vi "Mpemba1_QPDcali.vi"() -> ()   [LabVIEW 2019]
uses:
  <vilib>/rvi/Emulation/niFpgaGetClockAttributes.vi
  <vilib>/rvi/Emulation/niFpgaSctlEmulationGetInTimedLoop.vi
  <vilib>/rvi/Emulation/niFpgaEmulationReportErrorSimple.vi
  <vilib>/rvi/eio/common/nirviEmuTemplateMethod_errors.vi
  <vilib>/rvi/Emulation/niFpgaCriticalErrorInLSC.vi
  <vilib>/rvi/eio/common/nirviEmuTemplatePropertySet_noerrors.vi
  <vilib>/rvi/Emulation/niFpgaProcessEmulError.vi
  <vilib>/rvi/occurrence/nirviWaitOnOccurrenceBase.vi
  <vilib>/rvi/Emulation/niFpgaEmulationIsFPGAContextNoSignature.vi
  <vilib>/rvi/errors/niFpgaSetErrorForExecOnDevCompSimple.vi
  <vilib>/rvi/eio/common/nirviEmuReportErrorAndStop.vi
  <vilib>/rvi/DataTransferAndStorage/Container/Common/niFpgaContainerGetUniqueNameForEmu.vi
  <vilib>/rvi/FIFO/Fifo_Resource/nirvififoEmulationSetSize.vi
  <vilib>/rvi/FIFO/Fifo_Resource/nirviFifoEmulationQueueMgr.vi
  <instcachedir>/0/nirviFifoEmulationQueueMgr_E5CAEC123FF24DC58D834DCA3CDAA9B5.lvgen/nirviFifoEmulationQueueMgr_E5CAEC123FF24DC58D834DCA3CDAA9B5_001.vi
  <vilib>/Utility/error.llb/Clear Errors.vi
  <vilib>/rvi/FIFO/Fifo_Resource/nirvififoEmulationCreateLock.vi
  <vilib>/rvi/FIFO/Fifo_Resource/nirvififoEmulationObtainLock.vi
  <vilib>/rvi/FIFO/Fifo_Resource/nirvififoEmulationReleaseLock.vi
  <vilib>/rvi/errors/nirviReportUnexpectedCaseInternalError.vi
  <vilib>/rvi/errors/nirviReportUnexpectedCaseInternalError (U32).vi
  <vilib>/rvi/interface/RandomDataEmulation/niFpgaRandomDataHandleErrors.vi
  <vilib>/rvi/FIFO/Fifo_Resource/nirvififoEmulationDetermineInputValidOut.vi
  <vilib>/eio/EIONode/EIONode.xnode
  <vilib>/eio/EIOPropertyNode/EIOPropertyNode.xnode
  <vilib>/rvi/DataTransferAndStorage/Container/XNode/niFpgaContainer.xnode
  <vilib>/rvi/FIFO/Fifo_Resource/nirvififoEmulationRead.vi
  <vilib>/rvi/interface/RandomDataEmulation/nirviRandomDataFpgaReadWriteTemplate.vi
  <vilib>/rvi/FIFO/Fifo_Resource/nirvififoEmulationWrite.vi
  <vilib>/rvi/eio/common/nirviEmuTemplatePropertyGet_errors.vi
  <vilib>/rvi/eio/common/nirviEmuTemplatePropertyGet_noerrors.vi
  <vilib>/rvi/eio/common/nirviEmuTemplatePropertySet_errors.vi
panel:
  in  "Flat potential\nboundary":sgl=2.0 format="%#_13g"
  out "Protocol\nnumber":u32
  out "Protocol \nloops":i16
  out "Trigger":bool
  in  "hw cal\ntime":sgl=50.0
  in  "AOD_AO4 2":sgl
  in  "AOD_AO0 2":sgl
  in  "V_offset":sgl
  in  "Calibration":T1
  in  "Bias":sgl
  out "Time":i32
  in  "Fmax":sgl
  out "Fx out/Xcorr":sgl
  out "Xpot":sgl format="%.2f"
  in  "Temp":i8(ring) items=["Cold", "Warm", "Hot"]
  in  "cdfnorm":sgl
  out "Saveloop":u32
  in  "Enum":T2(ring)
  in  "MobX(px/V)":sgl
  in  "1/Xcali":sgl
  in  "Feedback parameters":T3
  in  "DX":sgl
  in  "DW":cluster{"xm":sgl, "Eb":sgl, "Tau":sgl, "dE":sgl}={"xm"=0.0, "Eb"=0.0, "Tau"=50.0, "dE"=0.0}
  in  "Xmean":sgl
  in  "Calibration ON/OFF":bool
  in  "Frequency":u32=100000
  in  "wait time":sgl=35.0
  in  "Triangle wave":T4={"signal offset_X"=5.0, "Scale X"=0.0, "signal offset_Y"=5.0, "Scale Y"=0.0, "Phase Shift"=30}
  in  "Xoffset":sgl
  in  "Yoffset":sgl
  in  "sum_offset":sgl
  in  "Normalize signal":bool=TRUE
  in  "FB Time":u8=5 caption="Feedback loop time"
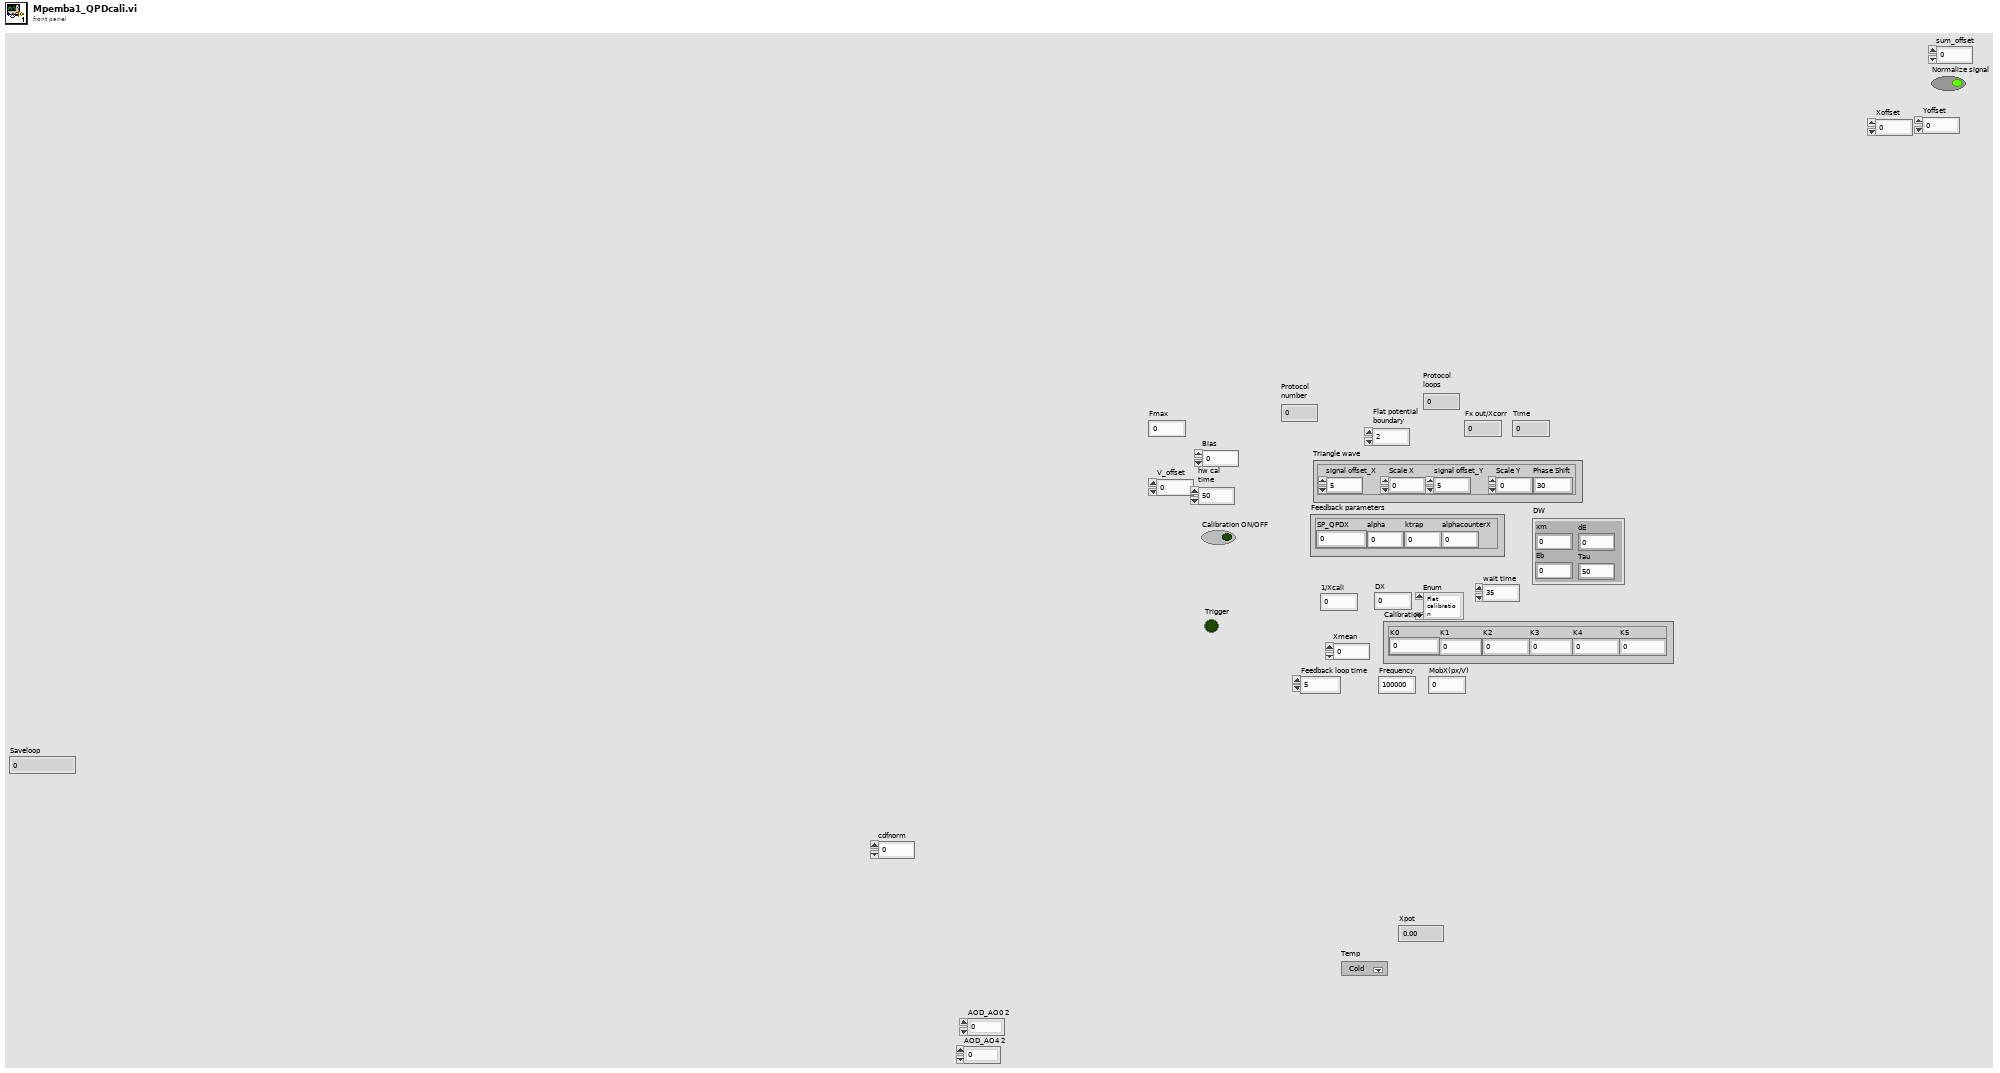
[diagram p1: front panel]
types:
  T1 = cluster{"K0":sgl, "K1":sgl, "K2":sgl, "K3":sgl, "K4":sgl, "K5":sgl}
  T2 = enum8{"Flat calibration", "Flat cal w drift corr", "No FB", "FB"}
  T3 = cluster{"SP_QPDX":sgl, "alpha":sgl, "ktrap":sgl, "alphacounterX":sgl}
  T4 = cluster{"signal offset_X":sgl, "Scale X":sgl, "signal offset_Y":sgl, "Scale Y":sgl, "Phase Shift":u32}
  T5 = enum8{"+/- 10 V", "+/- 5 V", "+/- 2 V", "+/- 1 V"}
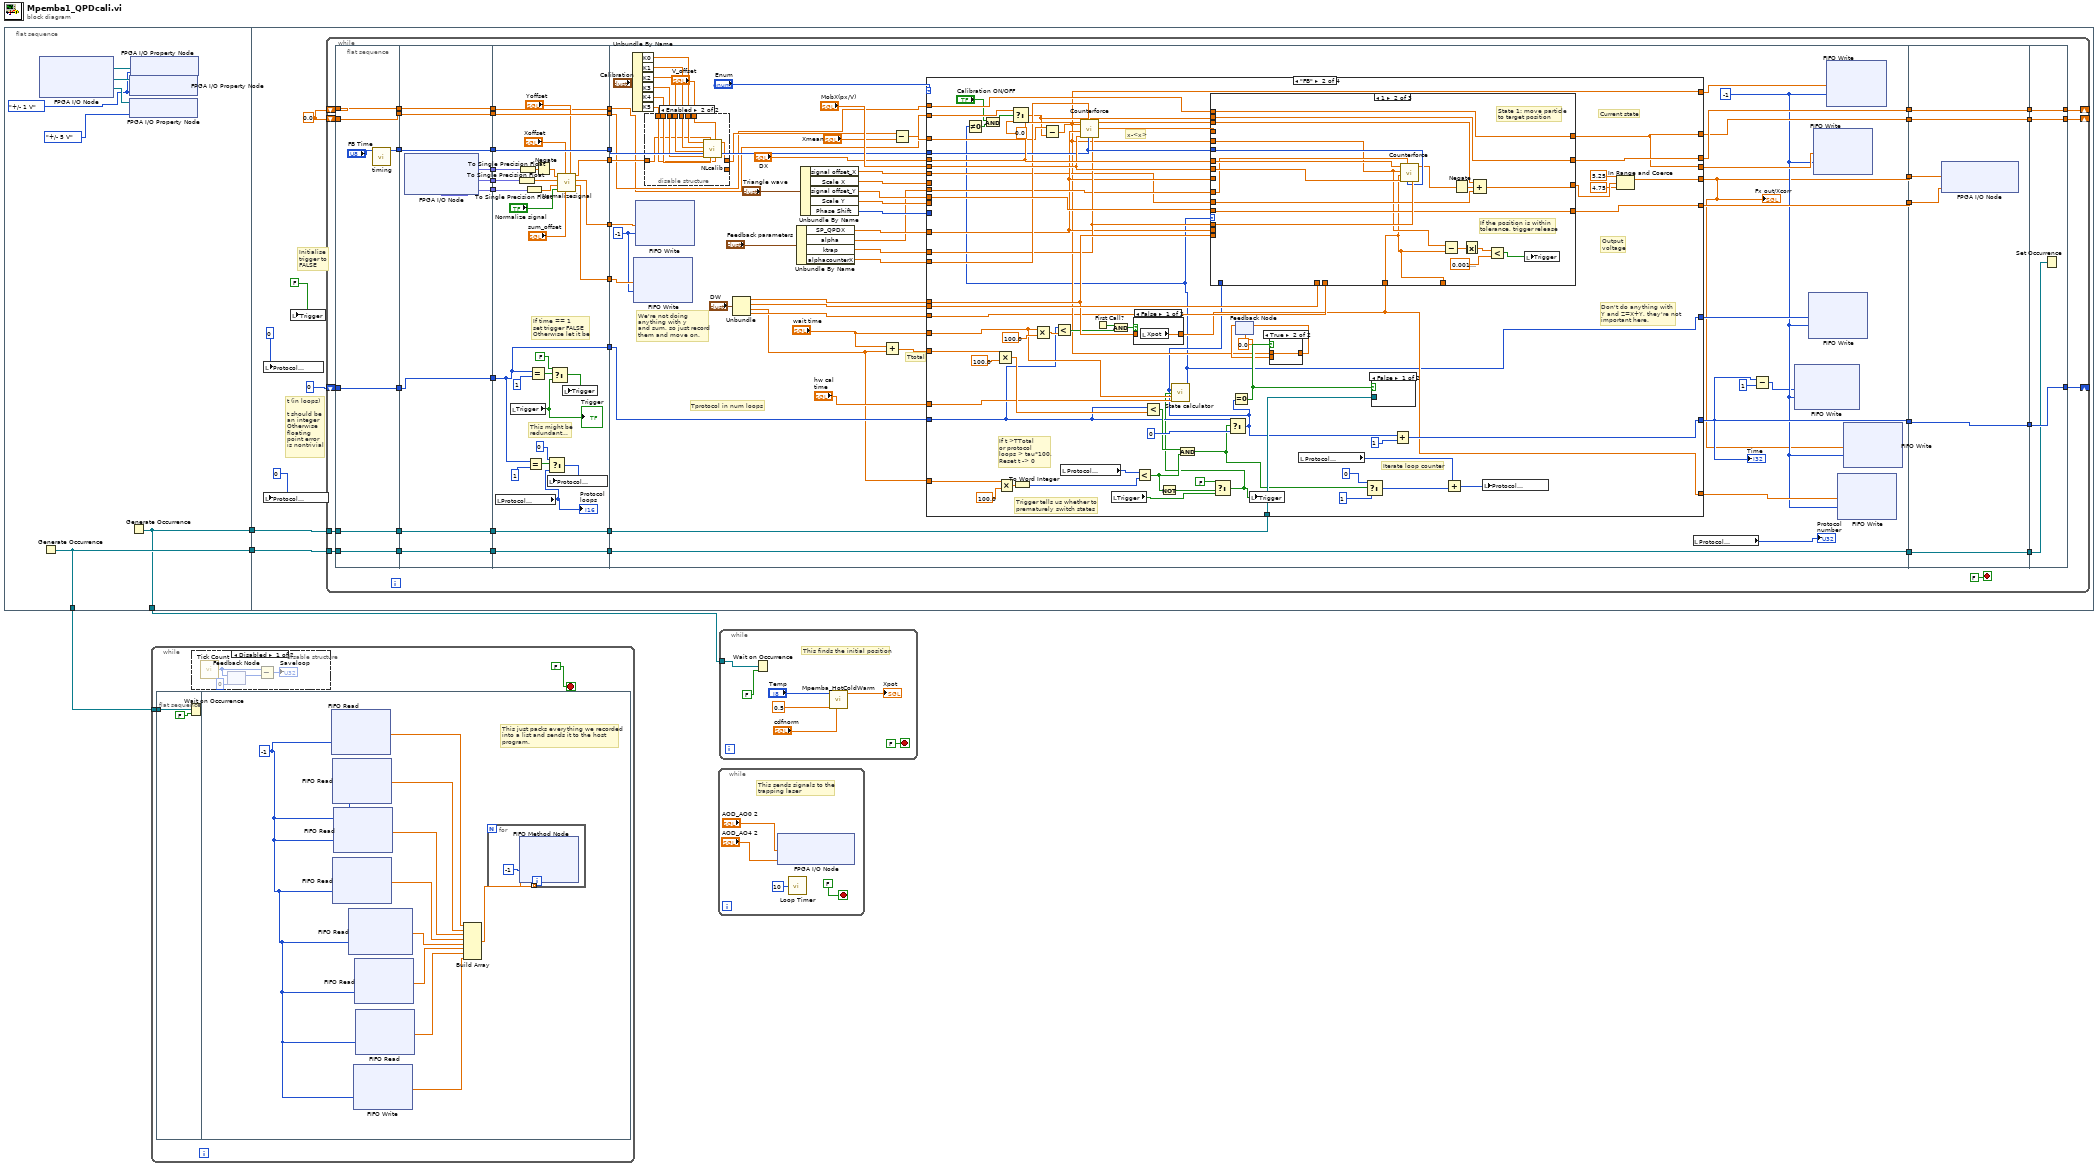
[diagram p0: block diagram]
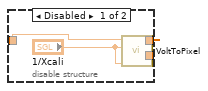
[diagram p2: hidden frame]
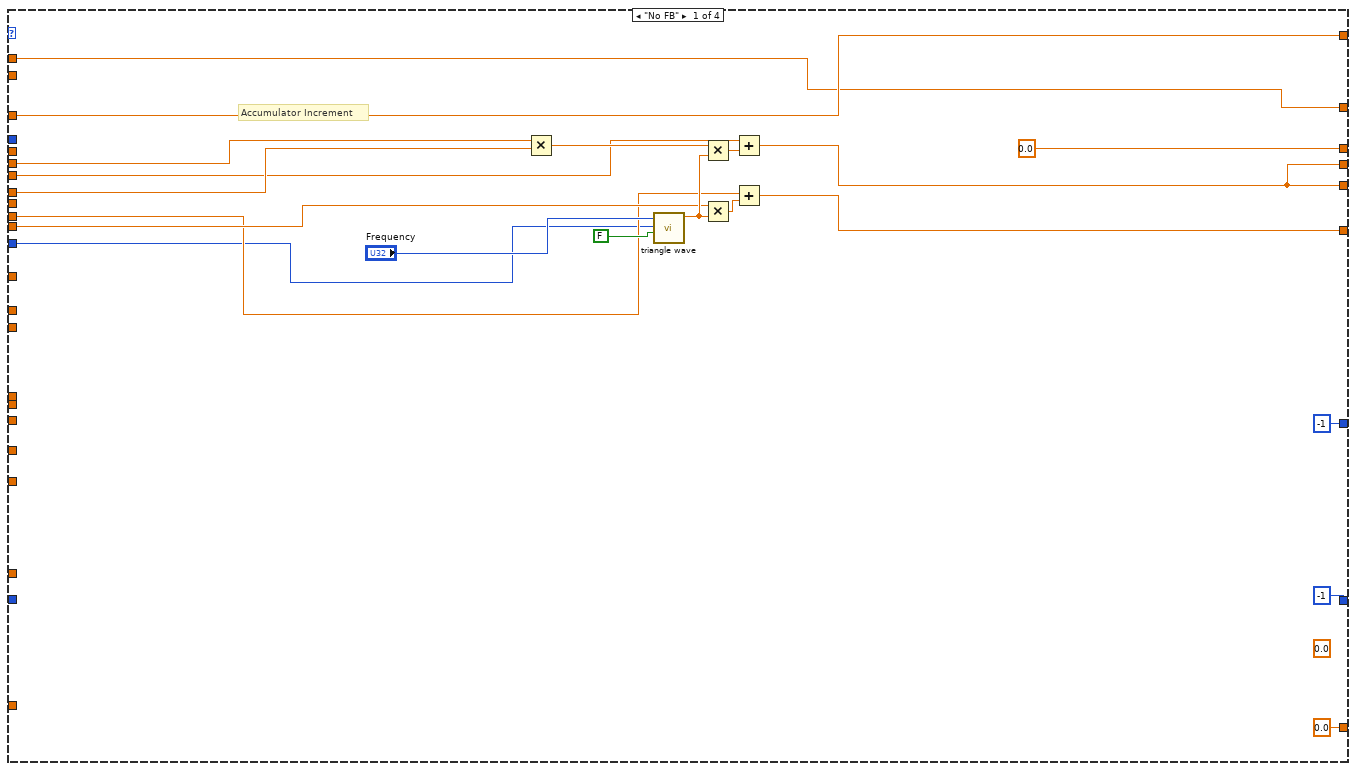
[diagram p3: hidden frame]
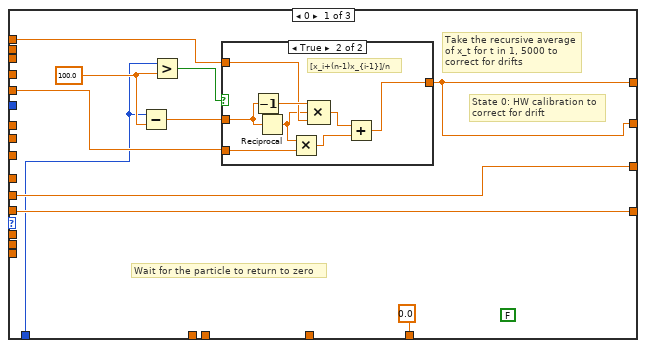
[diagram p4: hidden frame]
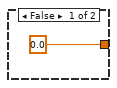
[diagram p5: hidden frame]
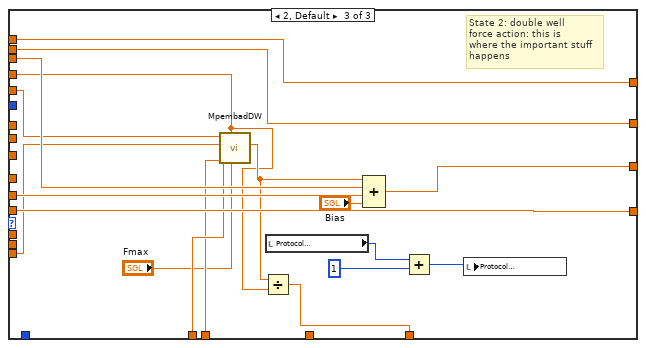
[diagram p6: hidden frame]
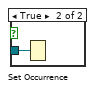
[diagram p7: hidden frame]
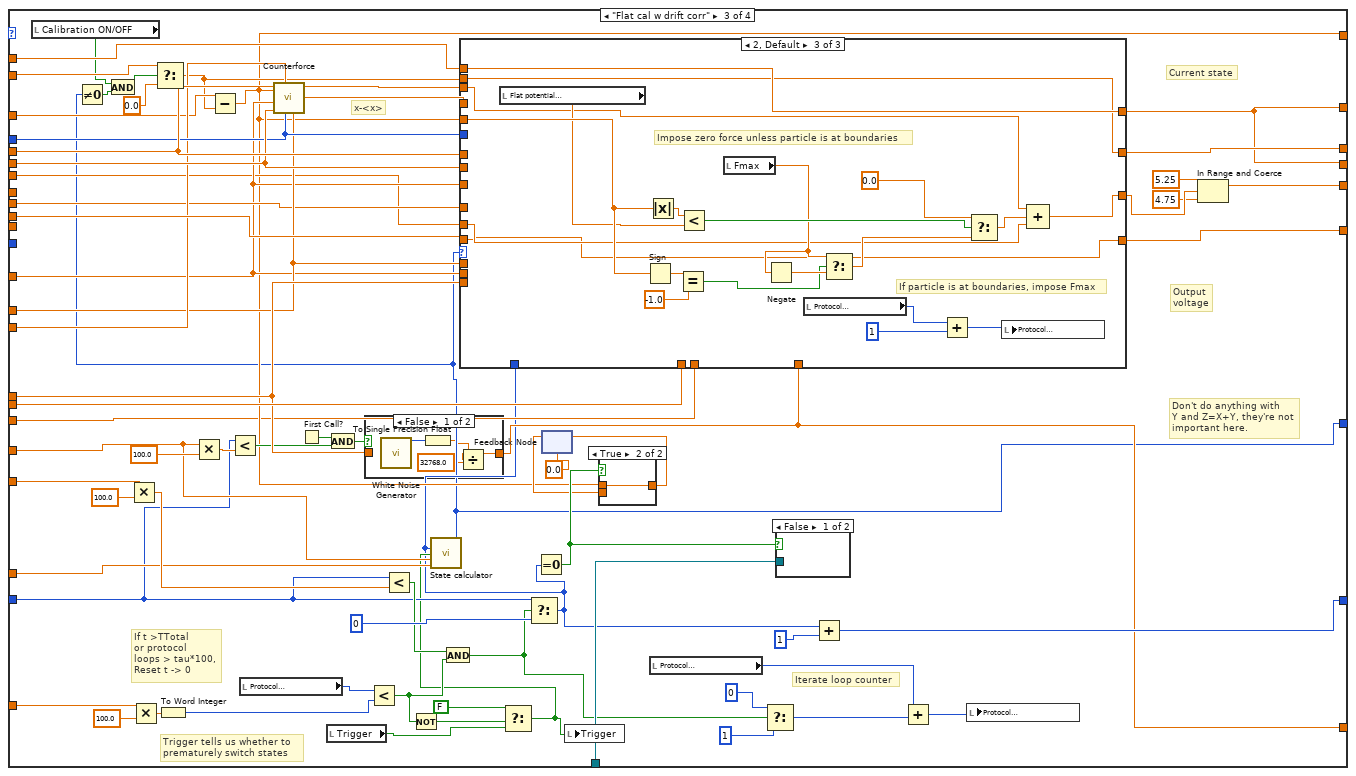
[diagram p10: hidden frame]
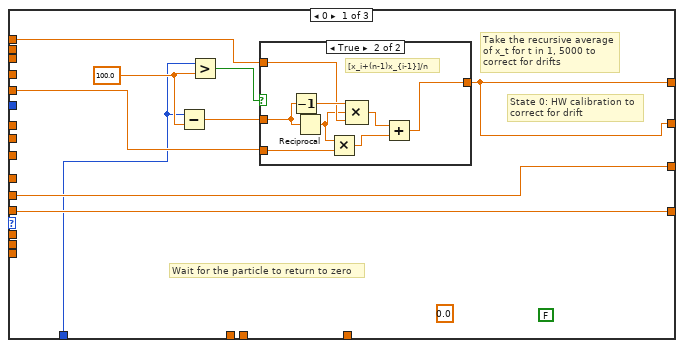
[diagram p11: hidden frame]
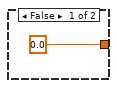
[diagram p12: hidden frame]
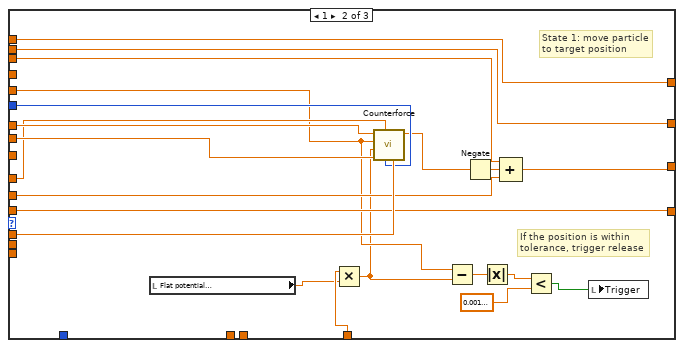
[diagram p13: hidden frame]
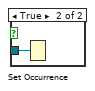
[diagram p14: hidden frame]
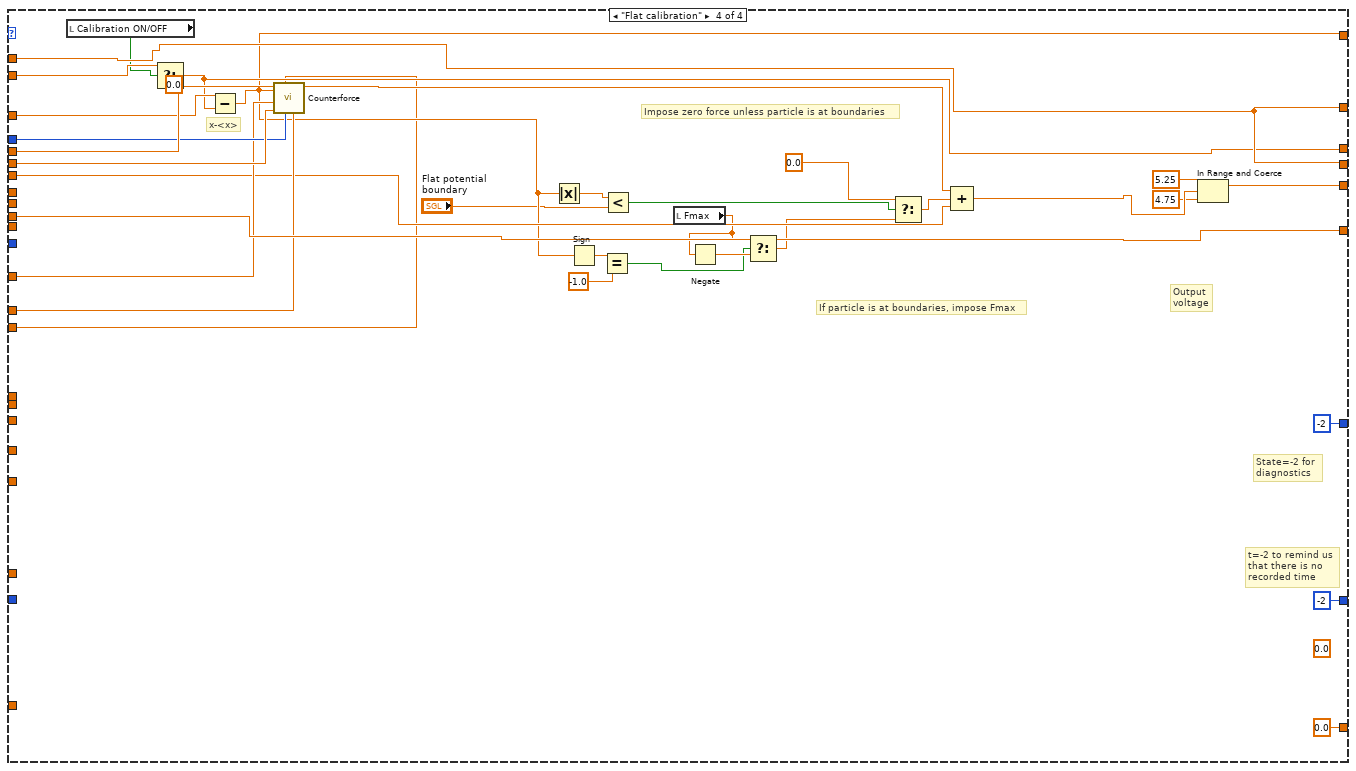
[diagram p17: hidden frame]
diagram:
  n1 = flat-sequence {
    tunnel: [w8] -> w2
    tunnel: [w7] -> w1
    tunnel: [w8] -> w4
    tunnel: [w7] -> w3
    tunnel: w2 -> [w18]
    tunnel: w1 -> [w17]
    frame #0 {
      w6 = T5."+/- 1 V" ("Voltage Range")
      n2 = xnode "FPGA I/O Node"() -> ("FPGA I/O Out"=w11:refnum<k21>, "FPGA I/O Out"=w9:refnum<k21>, "FPGA I/O Out"=w10:refnum<k21>)  [unwired: 3 in, 3 out]
      n3 = Generate Occurrence() -> (w8:refnum<k4>)
      n4 = xnode "FPGA I/O Property Node"("FPGA I/O In"=w9, "Voltage Range"=w6) -> ()  [unwired: 1 out]
      n5 = xnode "FPGA I/O Property Node"("FPGA I/O In"=w10, "Voltage Range"=T5."+/- 5 V") -> ()  [unwired: 1 out]
      n6 = Generate Occurrence() -> (w7:refnum<k4>)
      n7 = xnode "FPGA I/O Property Node"("FPGA I/O In"=w11, "Voltage Range"=w6) -> ()  [unwired: 1 out]
    }
    frame #1 {
      w16 = sgl 0.0
      # "t (in loops)\n\nt should be \nan integer\nOtherwise\nfloating\npoint error\nis nontrivial"
      # "Initialise\ntrigger to\nFALSE"
      n8 = local write "Protocol\nnumber"(u32 0 ("Protocol\nnumber")) -> ()
      n9 = local write "Protocol \nloops"(i16 0 ("Protocol loops")) -> ()
      n10 = local write "Trigger"(FALSE ("Trigger")) -> ()
      n11 = while {
        tunnel: w18 -> [w47]
        tunnel: w17 -> [w38]
        shift-right: [w35] -> _
        shift-left: w16 -> [w33]
        shift-right: [w28] -> _
        shift-left: w16 -> [w27]
        shift-right: [w19] -> _
        shift-left: i16 0 ("State") -> [w22]
        stop <- FALSE ("stop") stop-if-true
        n12 = flat-sequence {
          tunnel: [w67] -> w50
          tunnel: w47 -> [w66]
          tunnel: [w66] -> w46
          tunnel: [w65] -> w39
          tunnel: w38 -> [w65]
          tunnel: [w64] -> w34
          tunnel: w33 -> [w64]
          tunnel: w27 -> [w63]
          tunnel: [w63] -> w26
          tunnel: [w62] -> w23
          tunnel: w22 -> [w62]
          tunnel: [w77] -> w60
          tunnel: [w76] -> w58
          tunnel: [w75] -> w56
          tunnel: [w74] -> w51
          tunnel: w50 -> [w74]
          tunnel: w46 -> [w73]
          tunnel: [w73] -> w45
          tunnel: [w72] -> w40
          tunnel: w39 -> [w72]
          tunnel: w34 -> [w71]
          tunnel: [w71] -> w31
          tunnel: w26 -> [w70]
          tunnel: [w70] -> w25
          tunnel: w23 -> [w69]
          tunnel: [w69] -> w21
          tunnel: w60 -> [w91]
          tunnel: [w106] -> w59
          tunnel: w58 -> [w90]
          tunnel: [w105] -> w57
          tunnel: w56 -> [w89]
          tunnel: [w104] -> w55
          tunnel: [w107] -> w52
          tunnel: w51 -> [w107]
          tunnel: w45 -> [w103]
          tunnel: [w103] -> w44
          tunnel: [w102] -> w41
          tunnel: w40 -> [w102]
          tunnel: [w100] -> w32
          tunnel: w31 -> [w100]
          tunnel: w25 -> [w94]
          tunnel: [w94] -> w24
          tunnel: w21 -> [w78]
          tunnel: [w78] -> w20
          tunnel: w59 -> [w159]
          tunnel: w57 -> [w111]
          tunnel: w55 -> [w110]
          tunnel: [w112] -> w54
          tunnel: [w163] -> w53
          tunnel: w52 -> [w160]
          tunnel: [w119] -> w49
          tunnel: w44 -> [w152]
          tunnel: [w152] -> w42
          tunnel: w41 -> [w147]
          tunnel: [w115] -> w37
          tunnel: w32 -> [w145]
          tunnel: [w116] -> w30
          tunnel: w24 -> [w133]
          tunnel: w20 -> [w122]
          tunnel: w53 -> [w499]
          tunnel: w54 -> [w500]
          tunnel: w49 -> [w504]
          tunnel: [w504] -> w48
          tunnel: [w503] -> w43
          tunnel: w42 -> [w503]
          tunnel: w37 -> [w502]
          tunnel: [w502] -> w36
          tunnel: w30 -> [w501]
          tunnel: [w501] -> w29
          tunnel: w48 -> [w508]
          tunnel: [w508] -> w19
          tunnel: w43 -> [w507]
          tunnel: [w506] -> w35
          tunnel: w36 -> [w506]
          tunnel: w29 -> [w505]
          tunnel: [w505] -> w28
          frame #0 {
            n13 = call "timing.vi"("Feedback loop time"="FB Time") -> ("Feedback Loop time"=w67:u32)  [unwired: 10 in]
          }
          frame #1 {
            n14 = xnode "FPGA I/O Node"() -> ("Connector0/AI2"=w77:fxp<+/-,27,5>, "Connector0/AI4"=w76:fxp<+/-,27,5>, "Connector0/AI5"=w75:fxp<+/-,27,5>)  [unwired: 3 in, 3 out]
          }
          frame #2 {
            # "This might be\nredundant..."
            # "If time == 1\nset trigger FALSE\nOtherwise let it be"
            n15 = local read "Protocol \nloops"() -> (w80:i16)
            "Protocol \nloops" <- w80
            n16 = local read "Trigger"() -> (w84:bool)
            "Trigger" <- w84
            n17 = To Single Precision Float(number=w90) -> (single precision float=w96:sgl)
            n18 = To Single Precision Float(number=w91) -> (single precision float=w93:sgl)
            n19 = To Single Precision Float(number=w89) -> (single precision float=w95:sgl)
            n20 = Equal?(x=w78, y=i16 1) -> (x = y?=w82:bool)
            n21 = Equal?(x=w78, y=i16 1) -> (x = y?=w87:bool)
            n22 = Negate(x=w93) -> (-x=w92:sgl)
            n23 = Select(t=i16 0, s=w82, f=w80) -> (s? t:f=w81:i16)
            n24 = local write "Protocol \nloops"(w81) -> ()
            n25 = Select(t=FALSE, s=w87, f=w84) -> (s? t:f=w86:bool)
            n26 = call "Normalizesignal.vi"("Yoffset"="Yoffset", "sum_offset"="sum_offset", "Xoffset"="Xoffset", "Normalize signal"="Normalize signal", "Sum"=w95, "Y"=w96, "X"=w92) -> ("Sum"=w104:sgl, "Y"=w105:sgl, "X"=w106:sgl)  [unwired: 2 in]
            n27 = local write "Trigger"(w86) -> ()
          }
          frame #3 {
            w109 = -1 ("Timeout")
            w113 = -1 ("Timeout")
            # "We're not doing\nanything with y\nand sum, so just record\nthem and move on."
            # "Tprotocol in num loops"
            # "Ttotal"
            n28 = Unbundle By Name("Calibration") -> ("K0"=w130:sgl, "K1"=w129:sgl, "K2"=w128:sgl, "K3"=w127:sgl, "K4"=w126:sgl, "K5"=w125:sgl)
            n29 = xnode ("FIFO Write")("Element"=w110, "Timeout"=w109) -> ()  [unwired: 1 in, 2 out]
            n30 = xnode ("FIFO Write")("Element"=w111, "Timeout"=w109) -> ()  [unwired: 1 in, 2 out]
            n31 = disable-structure shown="Enabled" {
              disable-tunnel: w159 -> [w168 w170]
              disable-tunnel: [w166 _] -> _
              disable-tunnel: [w165 w169] -> w150
              disable-tunnel: "V_offset" -> [_ w177]
              disable-tunnel: w130 -> [_ w176]
              disable-tunnel: w129 -> [_ w175]
              disable-tunnel: w128 -> [_ w174]
              disable-tunnel: w127 -> [_ w173]
              disable-tunnel: w126 -> [_ w172]
              disable-tunnel: w125 -> [_ w171]
              frame Disabled {
                n32 = call "VoltToPixel.vi"("1/(QPDY/px)"="1/Xcali", "1/(QPDX/px)"="1/Xcali", "Normalized X"=w168) -> ("Ypx"=w166:sgl, "Xpx"=w165:sgl, "Normalized Y"=w167:sgl)  [unwired: 6 in]
              }
              frame Enabled {
                n33 = call "NLcalib.vi"("K5"=w171, "V_offset"=w177, "K4"=w172, "Volt QPD"=w170, "K3"=w173, "K2"=w174, "K1"=w175, "K0"=w176) -> ("pixels"=w169:sgl)  [unwired: 3 in]
              }
            }
            n34 = Unbundle("DW") -> ("xm"=w148:sgl, "Eb"=w157:sgl, "Tau"=w121:sgl, "dE"=w153:sgl)
            n35 = Unbundle By Name("Feedback parameters") -> ("SP_QPDX"=w137:sgl, "alpha"=w134:sgl, "ktrap"=w135:sgl, "alphacounterX"=w136:sgl)
            n36 = Unbundle By Name("Triangle wave") -> ("signal offset_X"=w141:sgl, "Scale X"=w143:sgl, "signal offset_Y"=w140:sgl, "Scale Y"=w142:sgl, "Phase Shift"=w139:u32)
            n37 = Add(x="wait time", y=w121) -> (x+y=w158:sgl)
            n38 = Subtract(x=w150, y="Xmean") -> (x-y=w155:sgl)
            n39 = case shown="\"FB\"" "Enum" {
              tunnel: w155 -> [w197 w236 w366 w483]
              tunnel: [w181 w250 w380 w494] -> w112
              tunnel: [w191 w244 w374 w493] -> w163
              tunnel: [w197 w234 w364 w481] -> w154
              tunnel: "MobX(px/V)" -> [w190 w263 w393 w497]
              tunnel: w160 -> [_ w251 w381 w495]
              tunnel: "DX" -> [_ w264 w394 w498]
              tunnel: w148 -> [_ w260 w390 _]
              tunnel: w157 -> [_ w265 w395 _]
              tunnel: w158 -> [_ w231 w361 _]
              tunnel: w153 -> [_ w204 w334 _]
              tunnel: w147 -> [_ w259 w389 _]
              tunnel: "wait time" -> [_ w219 w349 _]
              tunnel: [w189 w232 w362 w487] -> w115
              tunnel: w145 -> [w189 w240 w370 w487]
              tunnel: w143 -> [w187 _ _ _]
              tunnel: w142 -> [w186 _ _ _]
              tunnel: w141 -> [w185 w237 w367 w484]
              tunnel: w140 -> [w184 w249 w379 w493]
              tunnel: w139 -> [w183 _ _ _]
              tunnel: w137 -> [_ w241 w371 w488]
              tunnel: w136 -> [_ w248 w378 w480]
              tunnel: w135 -> [_ w247 w377 w492]
              tunnel: w134 -> [_ w246 w376 _]
              tunnel: [sgl 0.0 ("f") w233 w363 w482] -> w116
              tunnel: w133 -> [_ w238 w368 w485]
              tunnel: [w181 w232 w362 w487] -> w117
              tunnel: "hw cal\ntime" -> [_ w228 w358 _]
              tunnel: [i16 -1 ("f") w217 w347 i16 -2 ("f")] -> w119
              tunnel: [i16 -1 ("State") w201 w331 i16 -2 ("State")] -> w123
              tunnel: w122 -> [_ w218 w348 _]
              tunnel: w121 -> [_ w226 w356 _]
              tunnel: [sgl 0.0 ("dE") w203 w333 sgl 0.0 ("xm")] -> w114
              frame "No FB" {
                (unwired) sgl 0.0 ("DWvolt")
                # "Accumulator Increment"
                n40 = Multiply(x=w190, y=w187) -> (x*y=w195:sgl)
                n41 = call "triangle wave.vi"("Reset Accumulator_TW"=FALSE, "phase shift"=w183, "Frequency"="Frequency") -> ("Tri wave out"=w192:sgl)  [unwired: 8 in]
                n42 = Multiply(x=w195, y=w192) -> (x*y=w194:sgl)
                n43 = Multiply(x=w186, y=w192) -> (x*y=w196:sgl)
                n44 = Add(x=w185, y=w194) -> (x+y=w181:sgl)
                n45 = Add(x=w184, y=w196) -> (x+y=w191:sgl)
              }
              frame "FB" {
                # "Trigger tells us whether to \nprematurely switch states"
                # "If t >TTotal\nor protocol\nloops > tau*100,\nReset t -> 0"
                # "Don't do anything with\nY and Z=X+Y, they're not\nimportant here."
                # "x-<x>"
                # "Current state"
                # "Output\nvoltage"
                # "Iterate loop counter"
                n46 = Multiply(x=w231, y=sgl 100.0) -> (x*y=w229:sgl)
                n47 = Multiply(x=w226, y=sgl 100.0) -> (x*y=w224:sgl)
                n48 = To Word Integer(number=w224) -> (16bit integer=w223:i16)
                n49 = Multiply(x=w219, y=sgl 100.0) -> (x*y=w220:sgl)
                n50 = Less?(x=w218, y=w220) -> (x < y?=w253:bool)
                n51 = local read "Protocol \nloops"() -> (w227:i16)
                n52 = First Call?() -> (First Call?: T/F=w262:bool)
                n53 = local read "Trigger"() -> (w207:bool)
                n54 = And(x=w262, y=w253) -> (x .and. y?=w261:bool)
                n55 = case shown="False" w261 {
                  tunnel: [w326 w327] -> w203
                  tunnel: w260 -> [_ w327]
                  frame False {
                    n56 = local read "Xpot"() -> (w326:sgl)
                  }
                  frame True {
                  }
                }
                n57 = Less?(x=w227, y=w223) -> (x < y?=w209:bool)
                n58 = Less?(x=w218, y=w229) -> (x < y?=w222:bool)
                n59 = Not(x=w209) -> (.not. x?=w208:bool)
                n60 = And(x=w222, y=w209) -> (x .and. y?=w214:bool)
                n61 = Select(t=FALSE, s=w208, f=w207) -> (s? t:f=w205:bool)
                n62 = Select(t=w218, s=w214, f=i16 0) -> (s? t:f=w202:i16)
                n63 = call "State calculator.vi"("Current loop \nnumber"=w202, "Trigger"=w205, "wait time"=w219, "hw cal time"=w228) -> ("State"=w201:i8)  [unwired: 11 in]
                n64 = Not Equal To 0?(x=w201) -> (x != 0?=w200:bool)
                n65 = And(x="Calibration ON/OFF", y=w200) -> (x .and. y?=w198:bool)
                n66 = Select(t=w238, s=w198, f=sgl 0.0) -> (s? t:f=w235:sgl)
                n67 = Subtract(x=w236, y=w235) -> (x-y=w234:sgl)
                n68 = call "Counterforce.vi"("ktrap"=w247, "Ts"=w251, "alphacounterX"=w248, "mobX(px/V)"=w263, "SP_X"=w241, "Xpx"=w234, "Dx"=w264) -> ("ktrap*mob"=w257:sgl, "counter Force"=w258:sgl)  [unwired: 2 in, 1 out]
                n69 = case shown="1" w201 {
                  tunnel: w234 -> [w271 w292 w315]
                  tunnel: w264 -> [_ w304 _]
                  tunnel: w263 -> [_ w303 _]
                  tunnel: [w270 w302 w320] -> w245
                  tunnel: [w275 w299 w319] -> w244
                  tunnel: w247 -> [_ w300 _]
                  tunnel: w249 -> [w275 w299 w319]
                  tunnel: w237 -> [w270 w296 w322]
                  tunnel: w246 -> [_ w298 _]
                  tunnel: w260 -> [_ _ w314]
                  tunnel: w265 -> [_ _ w313]
                  tunnel: w258 -> [_ w297 w321]
                  tunnel: w257 -> [_ _ w306]
                  tunnel: w204 -> [_ _ w312]
                  tunnel: w241 -> [_ _ _]
                  tunnel: [w267 w294 w318] -> w232
                  tunnel: w240 -> [w272 w294 w318]
                  tunnel: w251 -> [_ w295 _]
                  tunnel: w203 -> [_ w286 _]
                  tunnel: w241 -> [_ _ _]
                  tunnel: [w267 w293 w317] -> w233
                  tunnel: w235 -> [_ w293 w317]
                  tunnel: [sgl 0.0 ("DWvolt") w286 w305] -> _
                  tunnel: w202 -> [w268 _ _]
                  frame 0 {
                    (unwired) FALSE
                    w276 = sgl 100.0 ("y")
                    # "Wait for the particle to return to zero"
                    # "State 0: HW calibration to\ncorrect for drift"
                    # "Take the recursive average\nof x_t for t in 1, 5000 to \ncorrect for drifts"
                    n70 = Subtract(x=w268, y=w276) -> (x-y=w273:sgl)
                    n71 = Greater?(x=w268, y=w276) -> (0:w274:bool)
                    n72 = case shown="True" w274 {
                      tunnel: [sgl 0.0 w279] -> w267
                      tunnel: w273 -> [_ w285]
                      tunnel: w272 -> [_ w283]
                      tunnel: w271 -> [_ w282]
                      frame False {
                      }
                      frame True {
                        # "[x_i+(n-1)x_{i-1}]/n"
                        n73 = Decrement(x=w285) -> (x-1=w284:sgl)
                        n74 = Reciprocal(x=w285) -> (1/x=w278:sgl)
                        n75 = Multiply(x=w278, y=w282) -> (x*y=w280:sgl)
                        n76 = Compound Arithmetic op=MULTIPLY(w284, w278, w283) -> (w281:sgl)
                        n77 = Add(x=w281, y=w280) -> (x+y=w279:sgl)
                      }
                    }
                  }
                  frame 1 {
                    # "State 1: move particle\nto target position"
                    # "If the position is within \ntolerance, trigger release"
                    n78 = call "Counterforce.vi"("ktrap"=w300, "Ts"=w295, "alphacounterX"=w298, "mobX(px/V)"=w303, "SP_X"=w286, "Xpx"=w292, "Dx"=w304) -> ("counter Force"=w287:sgl)  [unwired: 2 in, 2 out]
                    n79 = Subtract(x=w292, y=w286) -> (x-y=w291:sgl)
                    n80 = Negate(x=w287) -> (-x=w301:sgl)
                    n81 = Absolute Value(x=w291) -> (abs(x)=w290:sgl)
                    n82 = Compound Arithmetic op=ADD(w297, w301, w296) -> (w302:sgl)
                    n83 = Less?(x=w290, y=sgl 0.001) -> (x < y?=w288:bool)
                    n84 = local write "Trigger"(w288) -> ()
                  }
                  frame 2, Default {
                    # "State 2: double well \nforce action: this is\nwhere the important stuff\nhappens"
                    n85 = call "MpembadDW.vi"("Fmax"="Fmax", "ktrap*mob"=w306, "dE"=w312, "Eb"=w313, "Xm"=w314, "Xpos"=w315) -> ("DWvolt"=w307:sgl)  [unwired: 4 in, 1 out]
                    n86 = Divide(x=w307, y=w306) -> (x/y=w305:sgl)
                    n87 = local read "Protocol \nloops"() -> (w310:i16)
                    n88 = Compound Arithmetic op=ADD(w307, w321, w322, "Bias") -> (w320:sgl)
                    n89 = Add(x=w310, y=i16 1) -> (x+y=w308:i16)
                    n90 = local write "Protocol \nloops"(w308) -> ()
                  }
                }
                n91 = Equal To 0?(x=w202) -> (x = 0?=w256:bool)
                n92 = feedback #1(sgl 0.0) -> (w254:sgl)
                n93 = local write "Trigger"(w205) -> ()
                n94 = case shown="True" w256 {
                  tunnel: w234 -> [_ w325]
                  tunnel: [w324 w325] -> w255
                  tunnel: w254 -> [w324 _]
                  frame False {
                  }
                  frame True {
                  }
                }
                n95 = feedback-in #1(w255) -> ()
                n96 = local read "Protocol\nnumber"() -> (w215:u32)
                n97 = Select(t=i16 0, s=w214, f=i16 1) -> (s? t:f=w211:i16)
                n98 = case shown="False" w256 {
                  tunnel: w259 -> [_ w323]
                  frame False {
                  }
                  frame True {
                    n99 = Set Occurrence(w323) -> ()
                  }
                }
                n100 = Add(x=w202, y=i16 1) -> (x+y=w217:i16)
                n101 = Add(x=w215, y=w211) -> (x+y=w210:u32)
                n102 = local write "Protocol\nnumber"(w210) -> ()
                n103 = In Range and Coerce(upper limit=sgl 5.25, x=w245, lower limit=sgl 4.75) -> (coerced(x)=w250:sgl)  [unwired: 1 out]
              }
              frame "Flat cal w drift corr" {
                # "Trigger tells us whether to \nprematurely switch states"
                # "If t >TTotal\nor protocol\nloops > tau*100,\nReset t -> 0"
                # "Don't do anything with\nY and Z=X+Y, they're not\nimportant here."
                # "x-<x>"
                # "Current state"
                # "Output\nvoltage"
                # "Iterate loop counter"
                n104 = local read "Calibration ON/OFF"() -> (w328:bool)
                n105 = Multiply(x=w361, y=sgl 100.0) -> (x*y=w359:sgl)
                n106 = Multiply(x=w356, y=sgl 100.0) -> (x*y=w354:sgl)
                n107 = To Word Integer(number=w354) -> (16bit integer=w353:i16)
                n108 = Multiply(x=w349, y=sgl 100.0) -> (x*y=w350:sgl)
                n109 = Less?(x=w348, y=w350) -> (x < y?=w383:bool)
                n110 = local read "Protocol \nloops"() -> (w357:i16)
                n111 = First Call?() -> (First Call?: T/F=w392:bool)
                n112 = local read "Trigger"() -> (w337:bool)
                n113 = And(x=w392, y=w383) -> (x .and. y?=w391:bool)
                n114 = case shown="False" w391 {
                  tunnel: [w462 w464] -> w333
                  tunnel: w390 -> [_ w464]
                  frame False {
                    n115 = call "White Noise Generator"() -> ("white noise out"=w463:i16)  [unwired: 15 in]
                    n116 = To Single Precision Float(number=w463) -> (single precision float=w461:sgl)
                    n117 = Divide(x=w461, y=sgl 32768.0) -> (x/y=w462:sgl)
                  }
                  frame True {
                  }
                }
                n118 = Less?(x=w357, y=w353) -> (x < y?=w339:bool)
                n119 = Less?(x=w348, y=w359) -> (x < y?=w352:bool)
                n120 = Not(x=w339) -> (.not. x?=w338:bool)
                n121 = And(x=w352, y=w339) -> (x .and. y?=w344:bool)
                n122 = Select(t=FALSE, s=w338, f=w337) -> (s? t:f=w335:bool)
                n123 = Select(t=w348, s=w344, f=i16 0) -> (s? t:f=w332:i16)
                n124 = call "State calculator.vi"("Current loop \nnumber"=w332, "Trigger"=w335, "wait time"=w349, "hw cal time"=w358) -> ("State"=w331:i8)  [unwired: 11 in]
                n125 = Not Equal To 0?(x=w331) -> (x != 0?=w330:bool)
                n126 = And(x=w328, y=w330) -> (x .and. y?=w329:bool)
                n127 = Select(t=w368, s=w329, f=sgl 0.0) -> (s? t:f=w365:sgl)
                n128 = Subtract(x=w366, y=w365) -> (x-y=w364:sgl)
                n129 = call "Counterforce.vi"("ktrap"=w377, "Ts"=w381, "alphacounterX"=w378, "mobX(px/V)"=w393, "SP_X"=w371, "Xpx"=w364, "Dx"=w394) -> ("ktrap*mob"=w387:sgl, "counter Force"=w388:sgl)  [unwired: 2 in, 1 out]
                n130 = case shown="2, Default" w331 {
                  tunnel: w364 -> [w400 w423 w442]
                  tunnel: w394 -> [_ w435 _]
                  tunnel: w393 -> [_ w434 _]
                  tunnel: [w399 w433 w437] -> w375
                  tunnel: [w404 w430 w438] -> w374
                  tunnel: w377 -> [_ w431 _]
                  tunnel: w379 -> [w404 w430 w438]
                  tunnel: w367 -> [w399 w427 w440]
                  tunnel: w376 -> [_ w429 _]
                  tunnel: w390 -> [_ _ _]
                  tunnel: w395 -> [_ _ _]
                  tunnel: w388 -> [_ w428 w439]
                  tunnel: w387 -> [_ _ _]
                  tunnel: w334 -> [_ _ _]
                  tunnel: w371 -> [_ _ _]
                  tunnel: [w397 w425 w456] -> w362
                  tunnel: w370 -> [w401 w425 w456]
                  tunnel: w381 -> [_ w426 _]
                  tunnel: w333 -> [_ w416 _]
                  tunnel: w371 -> [_ _ _]
                  tunnel: [w397 w424 w436] -> w363
                  tunnel: w365 -> [_ w424 w436]
                  tunnel: w332 -> [w398 _ _]
                  frame 0 {
                    (unwired) sgl 0.0 ("DWvolt")
                    (unwired) FALSE
                    w405 = sgl 100.0 ("y")
                    # "Wait for the particle to return to zero"
                    # "State 0: HW calibration to\ncorrect for drift"
                    # "Take the recursive average\nof x_t for t in 1, 5000 to \ncorrect for drifts"
                    n131 = Subtract(x=w398, y=w405) -> (x-y=w402:sgl)
                    n132 = Greater?(x=w398, y=w405) -> (0:w403:bool)
                    n133 = case shown="True" w403 {
                      tunnel: [sgl 0.0 w408] -> w397
                      tunnel: w402 -> [_ w414]
                      tunnel: w401 -> [_ w412]
                      tunnel: w400 -> [_ w411]
                      frame False {
                      }
                      frame True {
                        # "[x_i+(n-1)x_{i-1}]/n"
                        n134 = Decrement(x=w414) -> (x-1=w413:sgl)
                        n135 = Reciprocal(x=w414) -> (1/x=w407:sgl)
                        n136 = Multiply(x=w407, y=w411) -> (x*y=w409:sgl)
                        n137 = Compound Arithmetic op=MULTIPLY(w413, w407, w412) -> (w410:sgl)
                        n138 = Add(x=w410, y=w409) -> (x+y=w408:sgl)
                      }
                    }
                  }
                  frame 1 {
                    # "State 1: move particle\nto target position"
                    # "If the position is within \ntolerance, trigger release"
                    n139 = local read "Flat potential\nboundary"() -> (w415:sgl)
                    n140 = Multiply(x=w416, y=w415) -> (x*y=w417:sgl)
                    n141 = call "Counterforce.vi"("ktrap"=w431, "Ts"=w426, "alphacounterX"=w429, "mobX(px/V)"=w434, "SP_X"=w417, "Xpx"=w423, "Dx"=w435) -> ("counter Force"=w418:sgl)  [unwired: 2 in, 2 out]
                    n142 = Subtract(x=w423, y=w417) -> (x-y=w422:sgl)
                    n143 = Negate(x=w418) -> (-x=w432:sgl)
                    n144 = Absolute Value(x=w422) -> (abs(x)=w421:sgl)
                    n145 = Compound Arithmetic op=ADD(w428, w432, w427) -> (w433:sgl)
                    n146 = Less?(x=w421, y=sgl 0.001) -> (x < y?=w419:bool)
                    n147 = local write "Trigger"(w419) -> ()
                  }
                  frame 2, Default {
                    # "If particle is at boundaries, impose Fmax"
                    # "Impose zero force unless particle is at boundaries"
                    n148 = local read "Flat potential\nboundary"() -> (w441:sgl)
                    n149 = Sign(1:w442) -> (0:w446:sgl)
                    n150 = Absolute Value(x=w442) -> (abs(x)=w452:sgl)
                    n151 = Equal?(x=w446, y=sgl -1.0) -> (x = y?=w444:bool)
                    n152 = Less?(x=w452, y=w441) -> (x < y?=w450:bool)
                    n153 = local read "Fmax"() -> (w449:sgl)
                    n154 = Negate(x=w449) -> (-x=w448:sgl)
                    n155 = local read "Protocol \nloops"() -> (w455:i16)
                    n156 = Select(t=w449, s=w444, f=w448) -> (s? t:f=w447:sgl)
                    n157 = Add(x=w455, y=i16 1) -> (x+y=w453:i16)
                    n158 = Select(t=sgl 0.0, s=w450, f=w447) -> (s? t:f=w451:sgl)
                    n159 = local write "Protocol \nloops"(w453) -> ()
                    n160 = Compound Arithmetic op=ADD(w439, w451, w440) -> (w437:sgl)
                  }
                }
                n161 = Equal To 0?(x=w332) -> (x = 0?=w386:bool)
                n162 = feedback #2(sgl 0.0) -> (w384:sgl)
                n163 = local write "Trigger"(w335) -> ()
                n164 = case shown="True" w386 {
                  tunnel: w364 -> [_ w459]
                  tunnel: [w458 w459] -> w385
                  tunnel: w384 -> [w458 _]
                  frame False {
                  }
                  frame True {
                  }
                }
                n165 = feedback-in #2(w385) -> ()
                n166 = local read "Protocol\nnumber"() -> (w345:u32)
                n167 = Select(t=i16 0, s=w344, f=i16 1) -> (s? t:f=w341:i16)
                n168 = case shown="False" w386 {
                  tunnel: w389 -> [_ w457]
                  frame False {
                  }
                  frame True {
                    n169 = Set Occurrence(w457) -> ()
                  }
                }
                n170 = Add(x=w332, y=i16 1) -> (x+y=w347:i16)
                n171 = Add(x=w345, y=w341) -> (x+y=w340:u32)
                n172 = local write "Protocol\nnumber"(w340) -> ()
                n173 = In Range and Coerce(upper limit=sgl 5.25, x=w375, lower limit=sgl 4.75) -> (coerced(x)=w380:sgl)  [unwired: 1 out]
              }
              frame "Flat calibration" {
                (unwired) sgl 0.0 ("xm")
                # "t=-2 to remind us\nthat there is no\nrecorded time"
                # "State=-2 for \ndiagnostics"
                # "If particle is at boundaries, impose Fmax"
                # "Impose zero force unless particle is at boundaries"
                # "x-<x>"
                # "Output\nvoltage"
                n174 = local read "Calibration ON/OFF"() -> (w479:bool)
                n175 = Select(t=w485, s=w479, f=sgl 0.0) -> (s? t:f=w482:sgl)
                n176 = Subtract(x=w483, y=w482) -> (x-y=w481:sgl)
                n177 = call "Counterforce.vi"("ktrap"=w492, "Ts"=w495, "alphacounterX"=w480, "mobX(px/V)"=w497, "SP_X"=w488, "Xpx"=w481, "Dx"=w498) -> ("counter Force"=w496:sgl)  [unwired: 2 in, 2 out]
                n178 = Absolute Value(x=w481) -> (abs(x)=w474:sgl)
                n179 = Sign(1:w481) -> (0:w468:sgl)
                n180 = Equal?(x=w468, y=sgl -1.0) -> (x = y?=w466:bool)
                n181 = Less?(x=w474, y="Flat potential\nboundary") -> (x < y?=w472:bool)
                n182 = local read "Fmax"() -> (w471:sgl)
                n183 = Negate(x=w471) -> (-x=w470:sgl)
                n184 = Select(t=w471, s=w466, f=w470) -> (s? t:f=w469:sgl)
                n185 = Select(t=sgl 0.0, s=w472, f=w469) -> (s? t:f=w473:sgl)
                n186 = Compound Arithmetic op=ADD(w496, w473, w484) -> (w491:sgl)
                n187 = In Range and Coerce(upper limit=sgl 5.25, x=w491, lower limit=sgl 4.75) -> (coerced(x)=w494:sgl)  [unwired: 1 out]
              }
            }
            "Fx out/Xcorr" <- w112
            "Time" <- w119
            n188 = local read "Protocol\nnumber"() -> (→"Protocol\nnumber":u32)
            n189 = Subtract(x=w119, y=i16 1) -> (x-y=w108:i16)
            n190 = xnode ("FIFO Write")("Element"=w108, "Timeout"=w113) -> ()  [unwired: 1 in, 2 out]
            n191 = xnode ("FIFO Write")("Element"=w123, "Timeout"=w113) -> ()  [unwired: 1 in, 2 out]
            n192 = xnode ("FIFO Write")("Element"=w117, "Timeout"=w113) -> ()  [unwired: 1 in, 2 out]
            n193 = xnode ("FIFO Write")("Element"=w154, "Timeout"=w113) -> ()  [unwired: 1 in, 2 out]
            n194 = xnode ("FIFO Write")("Element"=w114, "Timeout"=w113) -> ()  [unwired: 1 in, 2 out]
            n195 = xnode ("FIFO Write")("Element"=w112, "Timeout"=w113) -> ()  [unwired: 1 in, 2 out]
          }
          frame #4 {
            n196 = xnode "FPGA I/O Node"("Connector0/AO7"=w500, "Connector0/AO6"=w499) -> ()  [unwired: 2 in, 2 out]
          }
          frame #5 {
            n197 = Set Occurrence(w507) -> ()
          }
        }
      }
    }
  }
  n198 = while {
    tunnel: w4 -> [w509]
    stop <- FALSE stop-if-true
    n199 = flat-sequence {
      tunnel: w509 -> [w516]
      frame #0 {
        n200 = Wait on Occurrence(1:FALSE ("ignore previous (T)"), 2:w516) -> ()  [unwired: 1 in, 1 out]
      }
      frame #1 {
        w518 = -1 ("Timeout")
        # "This just packs everything we recorded\ninto a list and sends it to the host \nprogram."
        n201 = xnode ("FIFO Read")("Timeout"=w518) -> ("Element"=w524:sgl)  [unwired: 1 in, 2 out]
        n202 = xnode ("FIFO Read")("Timeout"=w518) -> ("Element"=w522:sgl)  [unwired: 1 in, 2 out]
        n203 = xnode ("FIFO Read")("Timeout"=w518) -> ("Element"=w523:sgl)  [unwired: 1 in, 2 out]
        n204 = xnode ("FIFO Read")("Timeout"=w518) -> ("Element"=w521:sgl)  [unwired: 1 in, 2 out]
        n205 = xnode ("FIFO Read")("Timeout"=w518) -> ("Element"=w525:sgl)  [unwired: 1 in, 2 out]
        n206 = xnode ("FIFO Write")("Timeout"=w518) -> ("Element"=w517:sgl)  [unwired: 1 in, 2 out]
        n207 = xnode ("FIFO Read")("Timeout"=w518) -> ("Element"=w520:sgl)  [unwired: 1 in, 2 out]
        n208 = xnode ("FIFO Read")("Timeout"=w518) -> ("Element"=w519:sgl)  [unwired: 1 in, 2 out]
        n209 = Build Array(w524, w522, w521, w523, w525, w520, w519, w517) -> (w526:sgl[])
        n210 = for {
          tunnel: w526 -> [w528] mode=indexing
          n211 = xnode ("FIFO Method Node")("Element"=w528, "Timeout"=-1) -> ()  [unwired: 1 in, 2 out]
        }
      }
    }
    n212 = disable-structure shown="Disabled" {
      frame Disabled {
        n213 = call "Tick Count"() -> ("Tick Count(uSec)"=w514:u32)
        n214 = feedback #3(u32 0 ("Tick Count(uSec)")) -> (w513:u32)
        n215 = feedback-in #3(w514) -> ()
        n216 = Subtract(x=w514, y=w513) -> (x-y=→"Saveloop":u32)
      }
      frame Enabled {
      }
    }
  }
  n217 = while {
    stop <- FALSE stop-if-true
    # "This sends signals to the \ntrapping laser"
    n218 = xnode "FPGA I/O Node"("Connector0/AO0"="AOD_AO0 2", "Connector0/AO4"="AOD_AO4 2") -> ()  [unwired: 2 in, 2 out]
    n219 = call "Loop Timer"("Count(uSec)"=u8 10) -> ()  [unwired: 1 out]
  }
  n220 = while {
    tunnel: w3 -> [w538]
    stop <- FALSE ("stop") stop-if-true
    # "This finds the initial position"
    n221 = Wait on Occurrence(1:FALSE ("ignore previous (T)"), 2:w538) -> ()  [unwired: 1 in, 1 out]
    n222 = call "Mpemba_HotColdWarm.vi"("RN"="cdfnorm", "X0"=sgl 0.5, "Ring"="Temp") -> ("Xpot"=→"Xpot":sgl)  [unwired: 8 in]
  }
